vi "MB Read Hold Register.vi"(8 "error in":errorcluster, 9 "Key":string, 11 "Devices":T1) -> (0 "error out":errorcluster, 2 "Register value":u16, 3 "Devices out":T1)   [LabVIEW 2021]
uses:
  <vilib>/NI/Modbus Library/API/Master/Modbus Master.lvclass
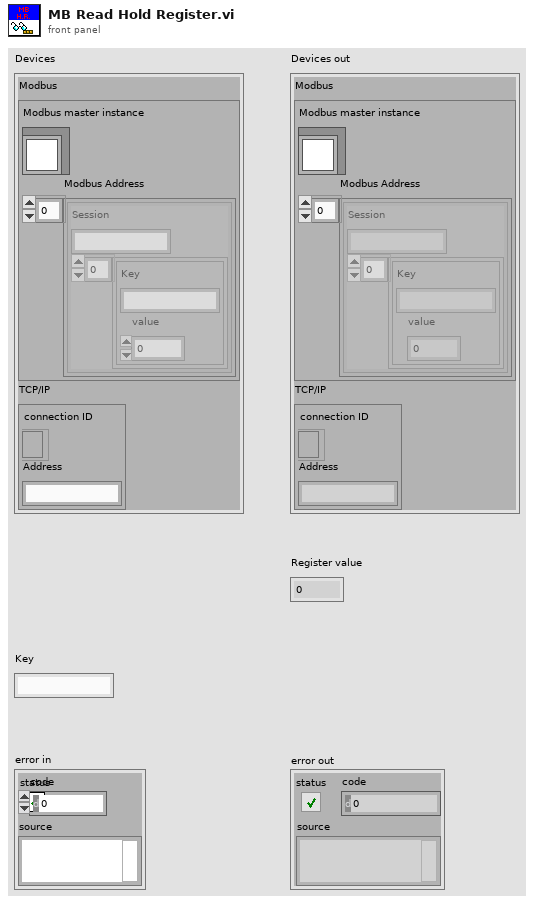
[diagram p1: front panel]
types:
  T1 = cluster{"Modbus":cluster{"Modbus master instance":refnum<class "Modbus Master.lvclass">, "Modbus Address":cluster{"Session":string, cluster{"Key":string, "value":u32}[]}[]}, "TCP/IP":cluster{"connection ID":refnum<k5>, "Address":string}}
  T2 = cluster{"Session":string, cluster{"Key":string, "value":u32}[]}[]
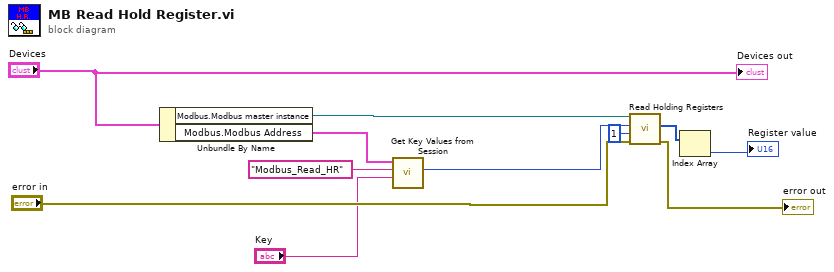
[diagram p0: block diagram]
diagram:
  n1 = Unbundle By Name("Devices") -> ("Modbus.Modbus master instance"=w11:refnum<class "Modbus Master.lvclass">, "Modbus.Modbus Address"=w9:T2)
  n2 = call "Get Key Values from Session.vi"("Key"="Key", "Session"="Modbus_Read_HR", "Ini File"=w9) -> ("Search Key Value"=w1:u32)  [unwired: 6 in, 2 out]
  n3 = call-dynamic "Read Holding Registers.vi"("error in"="error in", "number of inputs"=u16 1, "starting address"=w1, "Modbus master in"=w11) -> ("error out"=→"error out":errorcluster, "register values"=w5:u16[])  [unwired: 5 in, 1 out]
  n4 = Index Array(array=w5) -> (element=→"Register value":u16)  [unwired: 1 in]
  "Devices out" <- "Devices"
